vi "Prepare Paths For Expiration Check.vi"(0 "Scalar SA Path Group in":refnum<class "SA 18GHz Path Group.lvclass">, 5 "TSM Context":T1, 11 "error in (no error)":errorcluster) -> (4 "Scalar SA Path Group out":refnum<class "SA 18GHz Path Group.lvclass">, 15 "error out":errorcluster)   [LabVIEW 2023, in "RFFixtureCharact.RFPM.lvlib" / "SA 18GHz Path Group.lvclass"]
uses:
  SA 18GHz Path Group.lvclass
  C:/srd-semi-rfcal-software/AuxTools/STSRFFixtureCharactUtility/Source/Code Modules/Common/Base Classes/Path Group/Path Group.lvclass
  <vilib>/NI_TestStand_SemiconductorModule/NI_TestStand_Semiconductor_Module.lvlibp/PinMap/General/SemiconductorModuleContext.ctl
  Paths/SA Path/SA 18GHz Path.lvclass
  C:/srd-semi-rfcal-software/AuxTools/STSRFFixtureCharactUtility/Source/Code Modules/Common/Base Classes/Path/Path.lvclass
  Charact Result Accessor/Scalar/Scalar Charact Result Accessor.lvclass
  C:/srd-semi-rfcal-software/AuxTools/STSRFFixtureCharactUtility/Source/Code Modules/Fixture/RFPM/Charact Result Accessor/Base/Charact Result Accessor.lvclass
  C:/srd-semi-rfcal-software/AuxTools/STSRFFixtureCharactUtility/Source/Code Modules/Common/Result Accessor/Result Accessor.lvclass
  <vilib>/NI_TestStand_SemiconductorModule/NI_TestStand_Semiconductor_Module.lvlibp/PinMap/RF/RFmx/PinToNIRFmxSession.vi
  Common/Base Classes/Path/Path.lvclass
  Common/Result Accessor/Result Accessor.lvclass
  <vilib>/NI_TestStand_SemiconductorModule/NI_TestStand_Semiconductor_Module.lvlibp
  Common/Base Classes/Path Group/Path Group.lvclass
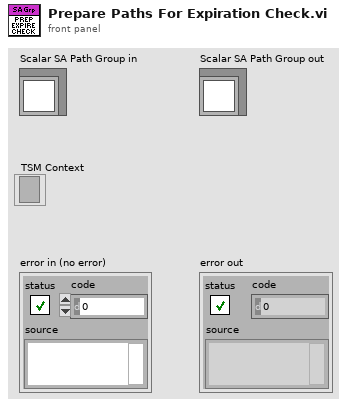
[diagram p1: front panel]
types:
  T1 = typedef "NI_TestStand_Semiconductor_Module.lvlibp/SemiconductorModuleContext.ctl" = refnum<k7>
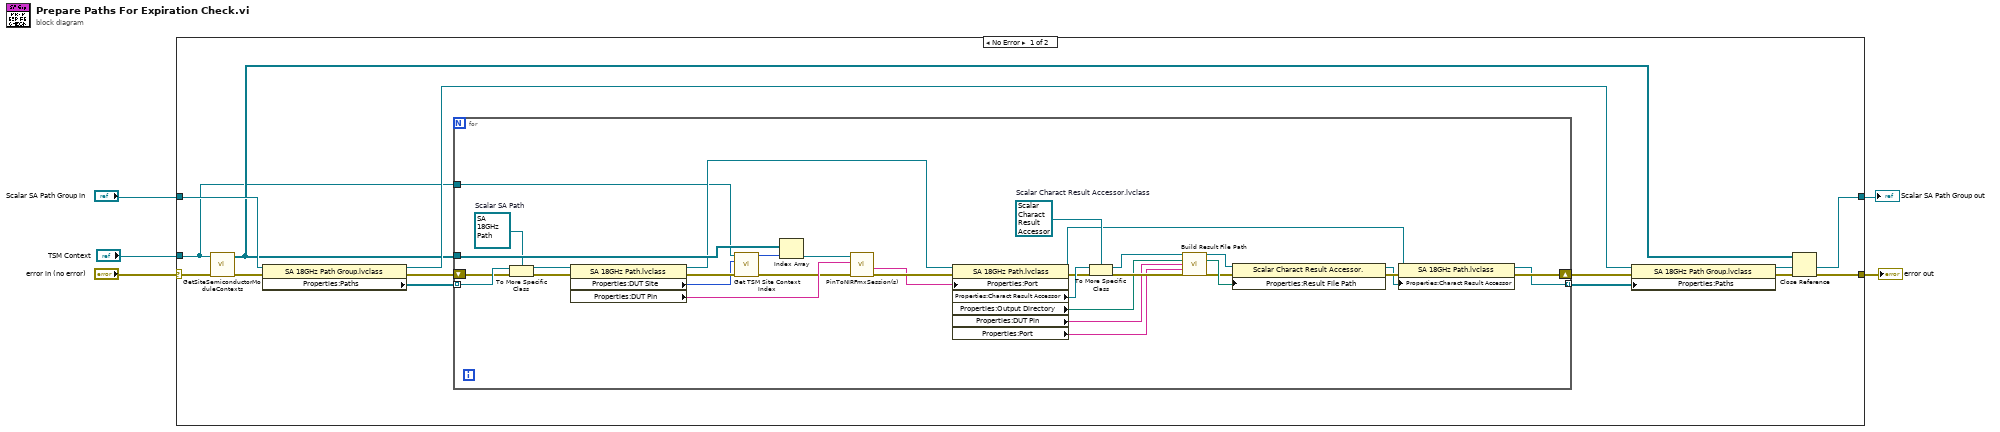
[diagram p0: block diagram]
diagram:
  n1 = case shown="No Error" "error in (no error)" {
    selector: "error in (no error)" -> [w10 w52]
    tunnel: "TSM Context" -> [w6 _]
    tunnel: "Scalar SA Path Group in" -> [w9 w51]
    tunnel: [w8 w52] -> w2
    tunnel: [w11 w51] -> w1
    frame No Error {
      n2 = call <vilib>:"GetSiteSemiconductorModuleContexts.vi"("error in (no error)"=w10, "Semiconductor Module Context"=w6) -> ("error out"=w15:errorcluster, "Site Semiconductor Module Contexts"=w7:T1[])  [unwired: 8 in]
      n3 = property class="SA 18GHz Path Group.lvclass"(reference=w9, error in=w15) -> (reference out=w13:refnum<class "SA 18GHz Path Group.lvclass">, error out=w17:errorcluster, "Properties:Paths"=w16:refnum<class "Path.lvclass">[])
      n4 = for {
        tunnel: w7 -> [w50]
        tunnel: w16 -> [w49] mode=indexing
        shift-right: [w31] -> w18
        shift-left: w17 -> [w45]
        tunnel: [w30] -> w12 mode=indexing
        tunnel: w6 -> [w37]
        w34 = refnum<class "Scalar Charact Result Accessor.lvclass"> refnum  # Scalar Charact Result Accessor.lvclass
        w46 = refnum<class "SA 18GHz Path.lvclass"> refnum  # Scalar SA Path
        n5 = To More Specific Class(target class=w46, reference=w49, error in=w45) -> (specific class reference=w47:refnum<class "SA 18GHz Path.lvclass">, error out=w44:errorcluster)
        n6 = property class="SA 18GHz Path.lvclass"(reference=w47, error in=w44) -> (reference out=w48:refnum<class "SA 18GHz Path.lvclass">, error out=w43:errorcluster, "Properties:DUT Site"=w36:i32, "Properties:DUT Pin"=w41:string)
        n7 = call "Get TSM Site Context Index.vi"("Semiconductor Module Context"=w37, "Site Number"=w36, "error in (no error)"=w43) -> ("index of Site TSM Context"=w35:i32, "error out"=w38:errorcluster)  [unwired: 11 in]
        n8 = Index Array(array=w50, index=w35) -> (element=w42:T1)
        n9 = call-poly <vilib>:"PinToNIRFmxSession(s).vi"("error in (no error)"=w38, "Pin"=w41, "Semiconductor Module Context"=w42) -> ("error out"=w40:errorcluster, "Port"=w39:string)  [unwired: 4 in, 3 out]
        n10 = property class="SA 18GHz Path.lvclass"(reference=w48, error in=w40, "Properties:Port"=w39) -> (reference out=w27:refnum<class "SA 18GHz Path.lvclass">, error out=w28:errorcluster, "Properties:Charact Result Accessor"=w29:refnum<class "Result Accessor.lvclass">, "Properties:Output Directory"=w21:path, "Properties:DUT Pin"=w20:string, "Properties:Port"=w19:string)
        n11 = To More Specific Class(target class=w34, reference=w29, error in=w28) -> (specific class reference=w26:refnum<class "Scalar Charact Result Accessor.lvclass">, error out=w23:errorcluster)
        n12 = call-dynamic "Build Result File Path.vi"("Charact Result Accessor in"=w26, "Output Directory"=w21, "Port 1"=w20, "Port 2"=w19, "error in"=w23) -> ("Charact Result Accessor out"=w25:refnum<class "Scalar Charact Result Accessor.lvclass">, "Result File Path"=w24:path, "error out"=w22:errorcluster)  [unwired: 8 in]
        n13 = property class="Scalar Charact Result Accessor."(reference=w25, error in=w22, "Properties:Result File Path"=w24) -> (reference out=w32:refnum<class "Scalar Charact Result Accessor.lvclass">, error out=w33:errorcluster)
        n14 = property class="SA 18GHz Path.lvclass"(reference=w27, error in=w33, "Properties:Charact Result Accessor"=w32) -> (reference out=w30:refnum<class "SA 18GHz Path.lvclass">, error out=w31:errorcluster)
      }
      n15 = property class="SA 18GHz Path Group.lvclass"(reference=w13, error in=w18, "Properties:Paths"=w12) -> (reference out=w11:refnum<class "SA 18GHz Path Group.lvclass">, error out=w14:errorcluster)
      n16 = Close Reference(reference=w7, error in (no error)=w14) -> (error out=w8:errorcluster)
    }
    frame Error {
    }
  }
  "Scalar SA Path Group out" <- w1
  "error out" <- w2
